vi "Discretization_DiscretizeABTaylor.vi"(6 "dT_Seconds":dbl, 7 "Inputs":i32, 9 "ContB":T1, 10 "ContA":T1, 11 "States":i32) -> (0 "Error":bool, 1 "DiscB":T1, 3 "DiscA":T1)   [LabVIEW 2019, in "Trajectory_Library.lvlib"]
doc: "Discretizes the given continuous A and B matrices.\n \nRather than solving a (States + Inputs) x (States + Inputs) matrix exponential like in DiscretizeAB(), we take advantage of the structure of the block matrix of A and B.\n\n 1) The exponential of A*t, which is only N x N, is relatively cheap. \n\n 2) The upper-right quarter of the (States + Inputs) x (States + Inputs) matrix, \n which we can approximate using a taylor series to several terms and still be \n substantially cheaper than taking the big exponential.\n\nInputs: \n - states -- the states of the system.\n - contA -- Continuous system matrix.\n - contB -- Continuous input matrix.\n - dtseconds -- Discretization timestep.\n\nOutputs:\n - DiscA -- Discretized A matrix\n - DiscB -- Discretized B matrix\n - Error -- If TRUE, an error occured."
uses:
  Trajectory_Library.lvlib
  <vilib>/Analysis/Matrix/NI_Matrix.lvlib
  <vilib>/Analysis/Matrix/Numeric/Add/Add - RM,RM.vi
  <vilib>/Analysis/Matrix/Numeric/Multiply/Multiply - RM,R.vi
  <vilib>/Analysis/NI_AALBase.lvlib
  <vilib>/Analysis/baseanly.llb/Real A x B.vi
  <vilib>/Analysis/Matrix/Datatypes/RealMatrix.ctl
panel:
  # "<States,States>"
  # "<States,Inputs>"
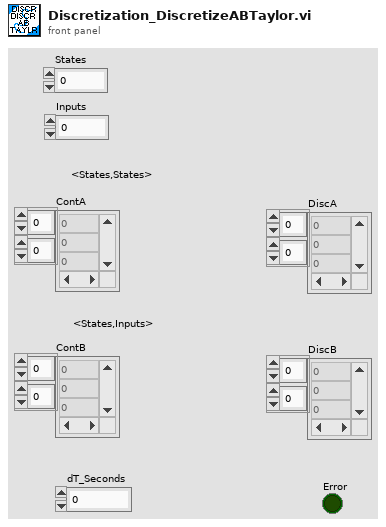
[diagram p1: front panel]
types:
  T1 = typedef "NI_Matrix.lvlib/RealMatrix.ctl" = dbl[][]
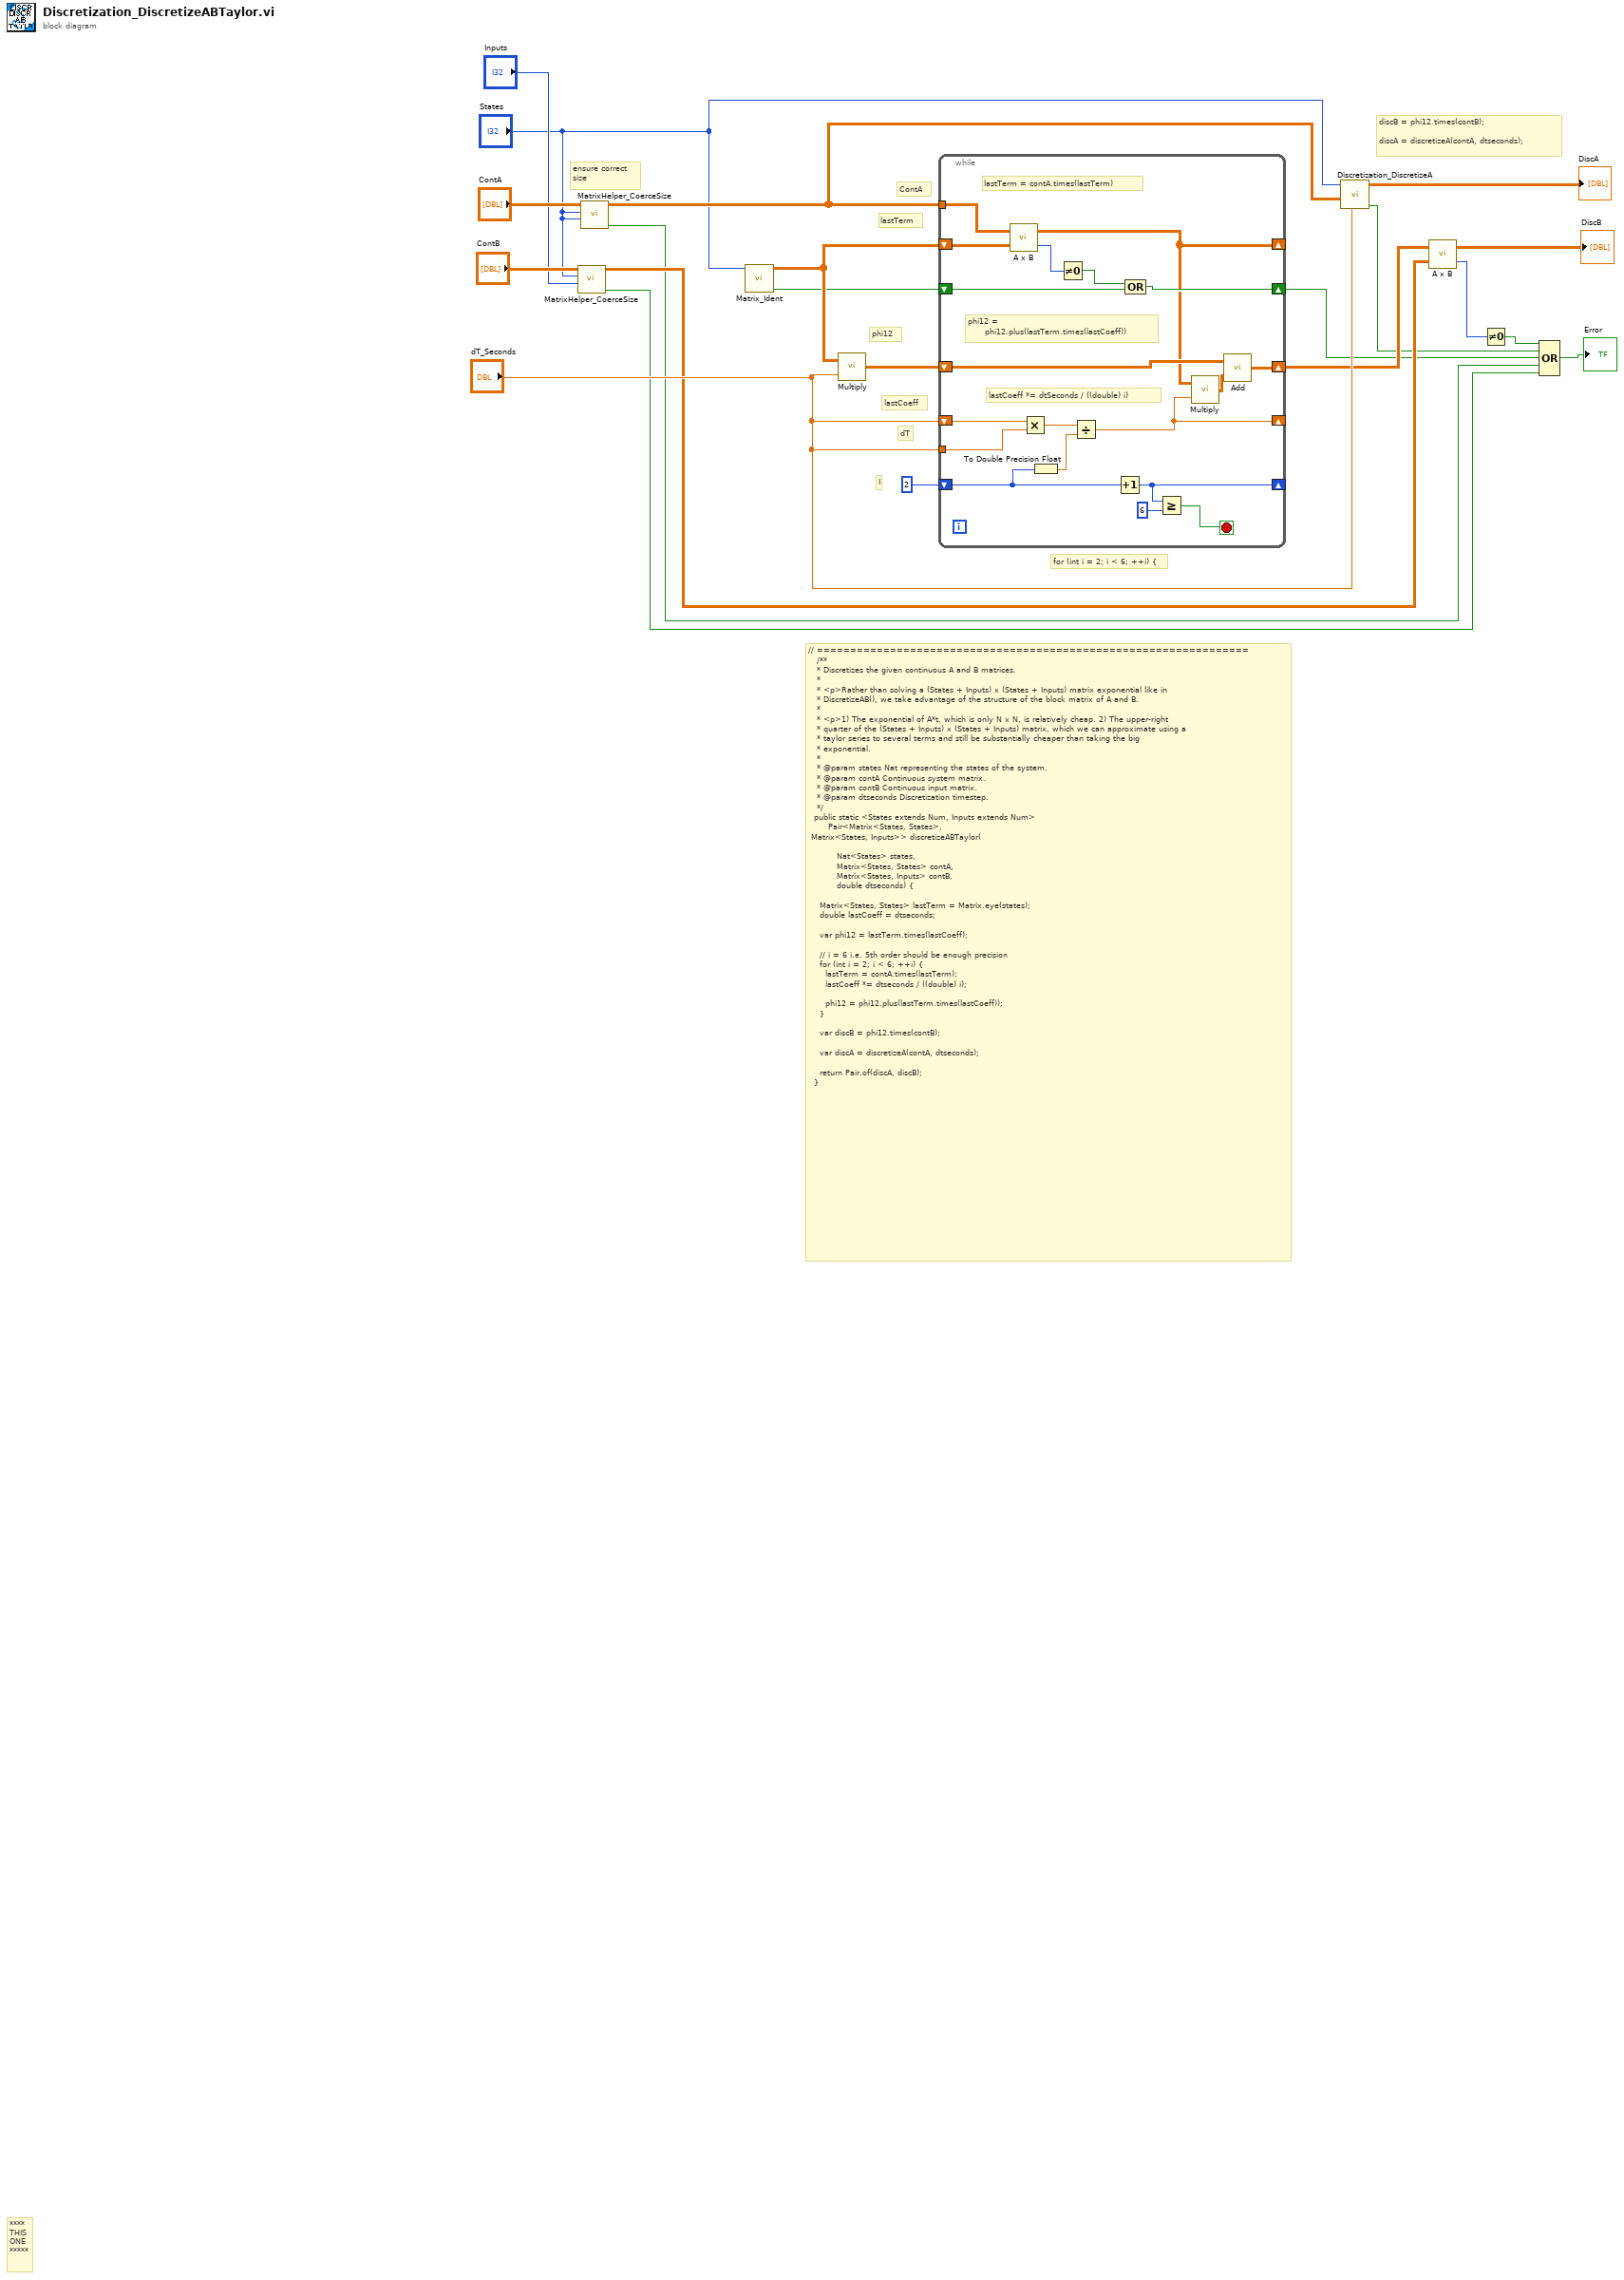
[diagram p0: block diagram]
diagram:
  # "// =================================================================\n   /**\n   * Discretizes the given continuous A and B matrices.\n   *\n   * <p>Rather than solving a (States + Inputs) x (States + Inputs) matrix exponential like in\n   * DiscretizeAB(), we take advantage of the structure of the block matrix of A and B.\n   *\n   * <p>1) The exponential of A*t, which is only N x N, is relatively cheap. 2) The upper-right\n   * quarter of the (States + Inputs) x (States + Inputs) matrix, which we can approximate using a\n   * taylor series to several terms and still be substantially cheaper than taking the big\n   * exponential.\n   *\n   * @param states Nat representing the states of the system.\n   * @param contA Continuous system matrix.\n   * @param contB Continuous input matrix.\n   * @param dtseconds Discretization timestep.\n   */\n  public static <States extends Num, Inputs extends Num>\n      \tPair<Matrix<States, States>, \n\tMatrix<States, Inputs>> discretizeABTaylor(\n\n          Nat<States> states,\n          Matrix<States, States> contA,\n          Matrix<States, Inputs> contB,\n          double dtseconds) {\n\n    Matrix<States, States> lastTerm = Matrix.eye(states);\n    double lastCoeff = dtseconds;\n\n    var phi12 = lastTerm.times(lastCoeff);\n\n    // i = 6 i.e. 5th order should be enough precision\n    for (int i = 2; i < 6; ++i) {\n      lastTerm = contA.times(lastTerm);\n      lastCoeff *= dtseconds / ((double) i);\n\n      phi12 = phi12.plus(lastTerm.times(lastCoeff));\n    }\n\n    var discB = phi12.times(contB);\n\n    var discA = discretizeA(contA, dtseconds);\n\n    return Pair.of(discA, discB);\n  }"
  # "discB = phi12.times(contB);\n\ndiscA = discretizeA(contA, dtseconds);"
  # "dT"
  # "ContA"
  # "for (int i = 2; i < 6; ++i) {"
  # "I"
  # "phi12"
  # "lastCoeff"
  # "lastTerm"
  # "ensure correct\nsize"
  # "****\nTHIS\nONE\n*****"
  n1 = call "MatrixHelper_CoerceSize.vi"("Columns"="Inputs", "Rows"="States", "input matrix"="ContB") -> ("Coerced"=w4:bool, "output matrix"=w8:T1)  [unwired: 7 in]
  n2 = call "MatrixHelper_CoerceSize.vi"("Columns"="States", "Rows"="States", "input matrix"="ContA") -> ("Coerced"=w3:bool, "output matrix"=w13:T1)  [unwired: 7 in]
  n3 = call "Matrix_Ident.vi"("Size"="States") -> ("Error"=w6:bool, "output matrix"=w7:T1)  [unwired: 9 in]
  n4 = call-poly <vilib>:"Multiply.vi"("Real Scalar c"="dT_Seconds", "Real Matrix A"=w7) -> ("A * c"=w20:T1)
  n5 = while {
    shift-right: [w23] -> _
    shift-left: w7 -> [w40]
    shift-right: [w35] -> _
    shift-left: "dT_Seconds" -> [w39]
    shift-right: [w30] -> _
    shift-left: 2 -> [w31]
    tunnel: w13 -> [w24]
    tunnel: "dT_Seconds" -> [w38]
    shift-right: [w32] -> w10
    shift-left: w20 -> [w34]
    shift-right: [w27] -> w2
    shift-left: w6 -> [w26]
    stop <- w28 stop-if-true
    # "lastTerm = contA.times(lastTerm)"
    # "phi12 = \n      phi12.plus(lastTerm.times(lastCoeff))"
    # "lastCoeff *= dtSeconds / ((double) i)"
    n6 = call-poly <vilib>:"A x B.vi"("B"=w40, "A"=w24) -> ("error"=w25:i32, "A x B"=w23:T1)
    n7 = Multiply(x=w39, y=w38) -> (x*y=w37:dbl)
    n8 = To Double Precision Float(number=w31) -> (double precision float=w36:dbl)
    n9 = Not Equal To 0?(x=w25) -> (x != 0?=w22:bool)
    n10 = Divide(x=w37, y=w36) -> (x/y=w35:dbl)
    n11 = Increment(x=w31) -> (x+1=w30:i32)
    n12 = Compound Arithmetic op=OR(w22, w26) -> (w27:bool)
    n13 = Greater Or Equal?(x=w30, y=6) -> (x >= y?=w28:bool)
    n14 = call-poly <vilib>:"Multiply.vi"("Real Scalar c"=w35, "Real Matrix A"=w23) -> ("A * c"=w33:T1)
    n15 = call-poly <vilib>:"Add.vi"("Real Matrix B"=w33, "Real Matrix A"=w34) -> ("A + B"=w32:T1)
  }
  n16 = call "Discretization_DiscretizeA.vi"("dT_Seconds"="dT_Seconds", "ContA"=w13, "States"="States") -> ("Error"=w1:bool, "DiscA"=→"DiscA":T1)  [unwired: 7 in]
  n17 = call-poly <vilib>:"A x B.vi"("B"=w8, "A"=w10) -> ("error"=w18:i32, "A x B"=→"DiscB":T1)
  n18 = Not Equal To 0?(x=w18) -> (x != 0?=w17:bool)
  n19 = Compound Arithmetic op=OR(w17, w1, w2, w3, w4) -> (→"Error":bool)
